vi "Annotation_Flip.vi"(7 "Flip":T3, 11 "Annotations (CWH)":T1[](array[typedef]) {"BBox"."x" format="%#_4p"; "BBox"."y" format="%#_4p"; "BBox"."w" format="%#_4p"; "BBox"."h" format="%#_4p"}) -> (3 "Annotations (CWH) out":T1[](array[typedef]) {"BBox"."x" format="%#_4p"; "BBox"."y" format="%#_4p"; "BBox"."w" format="%#_4p"; "BBox"."h" format="%#_4p"})   [LabVIEW 2020]
uses:
  Controls/Aug_Flip.ctl
  <vilib>/Ngene/Deep Learning Toolkit/Toolkit/NN_Data/API/Data/Detection_Types/NN_BBox_Annotation.ctl
  <vilib>/Ngene/Deep Learning Toolkit/Toolkit/NN_Data/API/Data/Detection_Types/NN_BBox.ctl
  <vilib>/Ngene/Deep Learning Toolkit/Toolkit/NN_Data/API/Data/Detection_Types/NN_BBox_Format_Conversion_Direction.ctl
  <vilib>/Ngene/Deep Learning Toolkit/Toolkit/Deep_Learning_Toolkit_by_Ngene.lvlib
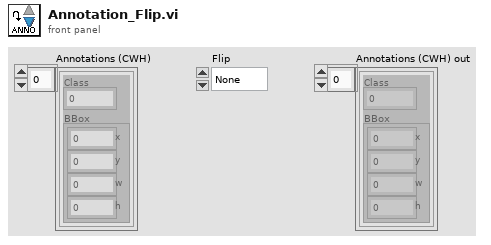
[diagram p1: front panel]
types:
  T1 = typedef "Deep_Learning_Toolkit_by_Ngene.lvlib/NN_BBox_Annotation.ctl" = cluster{"Class":i32, "BBox":T2}
  T2 = typedef "Deep_Learning_Toolkit_by_Ngene.lvlib/NN_BBox.ctl" = cluster{"x":sgl, "y":sgl, "w":sgl, "h":sgl}
  T3 = typedef "Aug_Flip.ctl" = enum16{"None", "Vertical", "Horizontal"}
  T4 = typedef "Deep_Learning_Toolkit_by_Ngene.lvlib/NN_BBox_Format_Conversion_Direction.ctl" = enum16{"SS_to_CWH", "CWH_to_SS"}
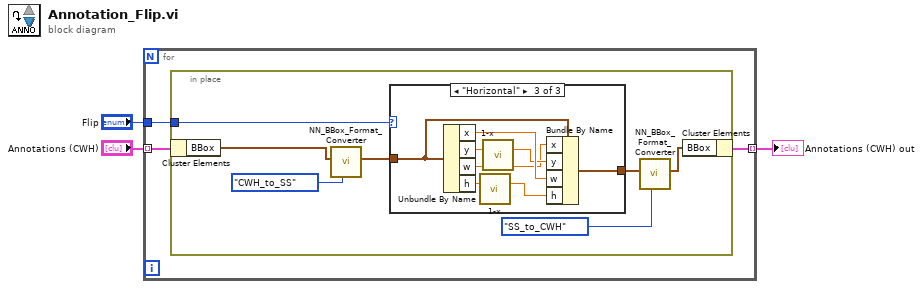
[diagram p0: block diagram]
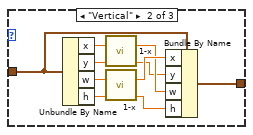
[diagram p3: hidden frame]
diagram:
  n1 = for {
    tunnel: "Annotations (CWH)" -> [w5] mode=indexing
    tunnel: "Flip" -> [w6]
    tunnel: [w4] -> w2 mode=indexing
    n2 = in-place {
      in-place-border: w6 -> [w7]
      n3 = in-place-cluster #1(w5) -> ("BBox"=w11:T2)
      n4 = call <vilib>:"NN_BBox_Format_Converter.vi"("Conversion_Direction"=NN_BBox_Format_Conversion_Direction."CWH_to_SS" ("Format_Transform"), "BBox in"=w11) -> ("BBox out"=w9:T2)  [unwired: 9 in]
      n5 = case shown="\"Horizontal\"" w7 {
        tunnel: w9 -> [w14 w16 w27]
        tunnel: [w14 w15 w26] -> w8
        frame "None", Default {
        }
        frame "Vertical" {
          n6 = Unbundle By Name(w16) -> ("x"=w20:sgl, "y"=w19:sgl, "w"=w18:sgl, "h"=w17:sgl)
          n7 = call "1-x.vi"("x"=w20) -> ("1-x"=w21:sgl)  [unwired: 14 in]
          n8 = call "1-x.vi"("x"=w18) -> ("1-x"=w22:sgl)  [unwired: 14 in]
          n9 = Bundle By Name(cluster=w16, "x"=w22, "y"=w19, "w"=w21, "h"=w17) -> (w15:T2)
        }
        frame "Horizontal" {
          n10 = Unbundle By Name(w27) -> ("x"=w30:sgl, "y"=w29:sgl, "w"=w23:sgl, "h"=w28:sgl)
          n11 = call "1-x.vi"("x"=w28) -> ("1-x"=w24:sgl)  [unwired: 14 in]
          n12 = call "1-x.vi"("x"=w29) -> ("1-x"=w25:sgl)  [unwired: 14 in]
          n13 = Bundle By Name(cluster=w27, "x"=w23, "y"=w25, "w"=w30, "h"=w24) -> (w26:T2)
        }
      }
      n14 = call <vilib>:"NN_BBox_Format_Converter.vi"("Conversion_Direction"=NN_BBox_Format_Conversion_Direction."SS_to_CWH" ("Format_Transform"), "BBox in"=w8) -> ("BBox out"=w10:T2)  [unwired: 9 in]
      n15 = in-place-cluster #1("BBox"=w10) -> (w4:T1)
    }
  }
  "Annotations (CWH) out" <- w2
